vi "afd11.vi"(4 "dpp":dbl, 5 "phase0,deg":dbl, 6 "Y":i16[](array[numeric]), 7 "afd_in":cluster{i16[], i32[]}[](array[cluster]), 8 "hist_in":cluster{i16[], i32[]}) -> (2 "afd_out":cluster{i16[], i32[]}[](array[cluster]), 3 "hist_out":cluster{i16[], i32[]})   [LabVIEW 2010]
panel:
  # "АФД как одномерный\nмассив гистограмм"
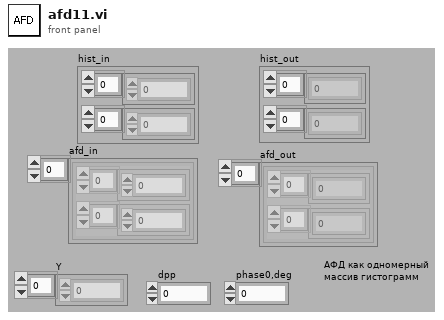
[diagram p1: front panel]
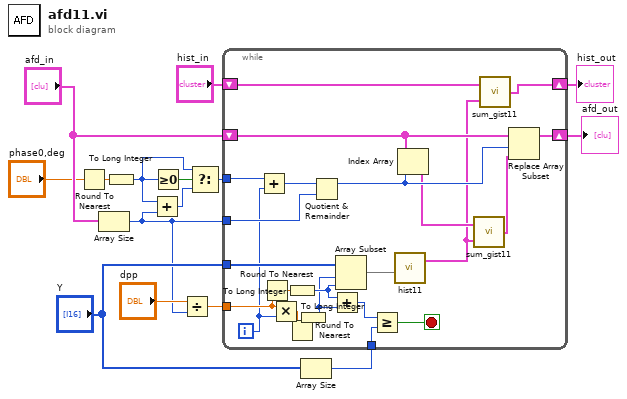
[diagram p0: block diagram]
diagram:
  n1 = Round To Nearest(number="phase0,deg") -> (nearest integer value=w2:dbl)
  n2 = Array Size(array="afd_in") -> (size(s)=w6:i32)
  n3 = To Long Integer(number=w2) -> (32bit integer=w1:i32)
  n4 = Add(x=w1, y=w6) -> (x+y=w10:i32)
  n5 = Greater Or Equal To 0?(x=w1) -> (x >= 0?=w12:bool)
  n6 = Divide(x="dpp", y=w6) -> (x/y=w7:dbl)
  n7 = Select(t=w1, s=w12, f=w10) -> (s? t:f=w11:i32)
  n8 = Array Size(array="Y") -> (size(s)=w14:i32)
  n9 = while {
    tunnel: "Y" -> [w34]
    tunnel: w7 -> [w37]
    tunnel: w14 -> [w30]
    tunnel: w6 -> [w27]
    shift-right: [w24] -> w15
    shift-left: "afd_in" -> [w25]
    tunnel: w11 -> [w21]
    shift-right: [w18] -> w5
    shift-left: "hist_in" -> [w17]
    i -> [w23]
    stop <- w29 stop-if-true
    n10 = Add(x=w21, y=w23) -> (x+y=w22:i32)
    n11 = Round To Nearest(number=w37) -> (nearest integer value=w36:dbl)
    n12 = Multiply(x=w37, y=w23) -> (x*y=w38:dbl)
    n13 = To Long Integer(number=w36) -> (32bit integer=w33:i32)
    n14 = Round To Nearest(number=w38) -> (nearest integer value=w35:dbl)
    n15 = To Long Integer(number=w35) -> (32bit integer=w32:i32)
    n16 = Quotient & Remainder(x=w22, y=w27) -> (x-y*floor(x/y)=w26:i32)  [unwired: 1 out]
    n17 = Add(x=w33, y=w32) -> (x+y=w31:i32)
    n18 = Array Subset(array=w34, index=w32, length=w33) -> (w28:i16[])
    n19 = Greater Or Equal?(x=w31, y=w30) -> (x >= y?=w29:bool)
    n20 = call "hist11.vi"("Y"=w28) -> ("hist"=w16:cluster{i16[], i32[]})  [unwired: 4 in]
    n21 = Index Array(array=w25, index=w26) -> (element=w20:cluster{i16[], i32[]})
    n22 = call "sum_gist11.vi"("hist2"=w16, "hist1"=w20) -> ("hist1+2"=w19:cluster{i16[], i32[]})
    n23 = call "sum_gist11.vi"("hist2"=w16, "hist1"=w17) -> ("hist1+2"=w18:cluster{i16[], i32[]})
    n24 = Replace Array Subset(array=w25, new element=w19, index=w26) -> (w24:cluster{i16[], i32[]}[])
  }
  "afd_out" <- w15
  "hist_out" <- w5
